vi "sort_property.vi"(6 "Property Order by Default":string[](array[string]), 8 "Sorting Method":u16, 9 "Array to Sort":string[](array[string]), 10 "Property":string[](array[string]), 11 "CmdInfo":T1(array[cluster])=[{"Property"="Arm Slope", "SCPI Command"=":ARM:START:SLOP POS|NEG", "Description"="", "Group"=""}, {"Property"="Arm Enum", "SCPI Command"=":ARM:START:SLOP OK|CANCLE", "Description"="", "Group"=""}]) -> (1 "Sorted Array":string[](array[string]))   [LabVIEW 2018]
doc: "Sort the properties. There are 3 kinds of sorting. When sorting method sets to 0, the properties will be sorted according to their ordir in source command file. When sorting method sets to 1, the properties will be sorted by property names. When sorting method sets to 2, the properties will be sorted by SCPI commands."
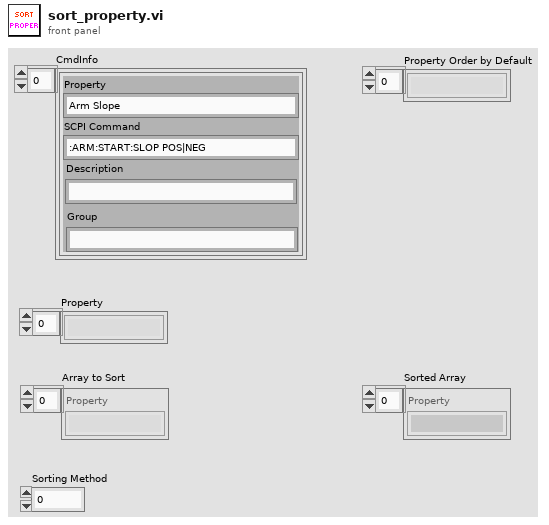
[diagram p1: front panel]
types:
  T1 = cluster{"Property":string, "SCPI Command":string, "Description":string, "Group":string}[]
  T2 = cluster{"SCPI Command":string, "Property":string}[]
  T3 = cluster{"SCPI Command":string, "Property":string}
  T4 = cluster{"Property":string, "SCPI Command":string, "Description":string, "Group":string}
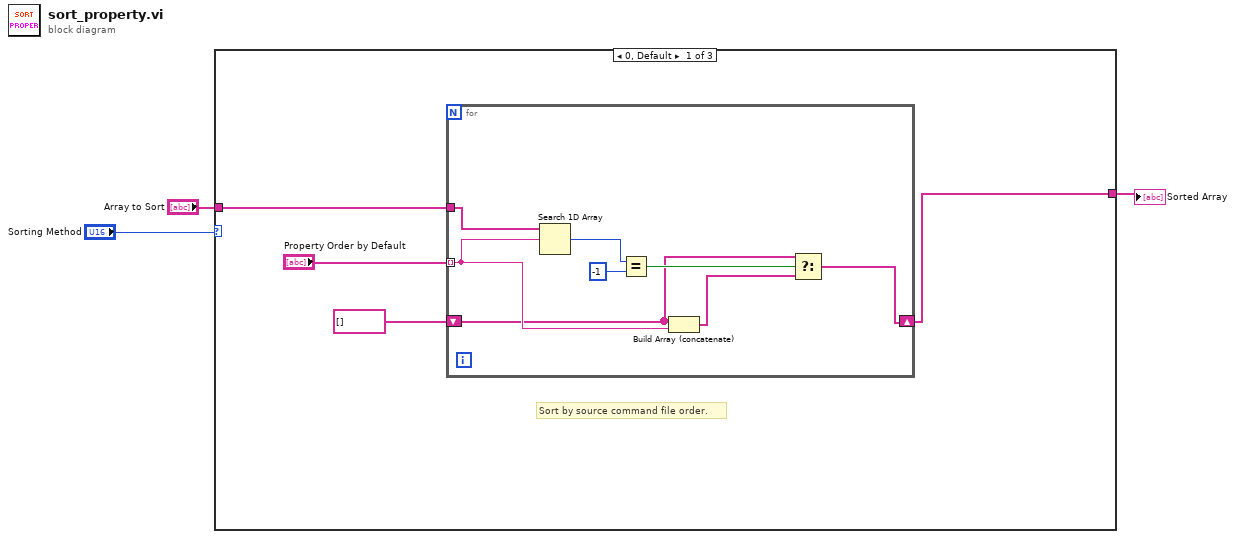
[diagram p0: block diagram]
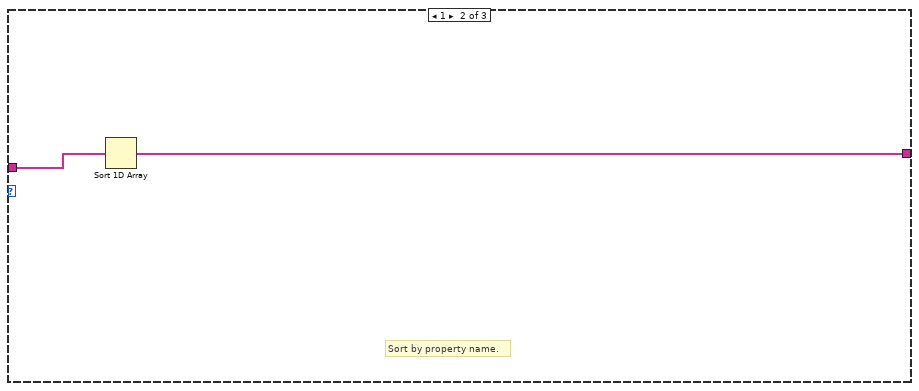
[diagram p2: hidden frame]
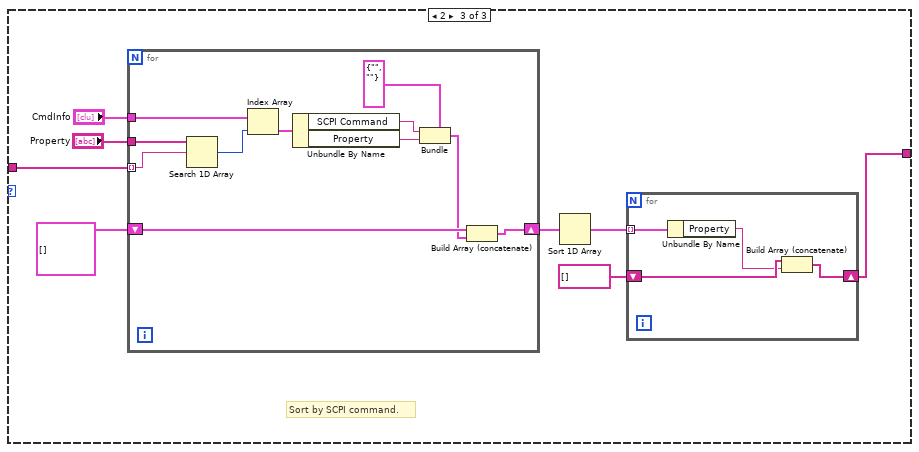
[diagram p3: hidden frame]
diagram:
  n1 = case shown="0, Default" "Sorting Method" {
    tunnel: "Array to Sort" -> [w6 w17 w22]
    tunnel: [w4 w16 w18] -> w1
    frame 0, Default {
      # "Sort by source command file order."
      n2 = for {
        tunnel: "Property Order by Default" -> [w10] mode=indexing
        tunnel: w6 -> [w15]
        shift-right: [w14] -> w4
        shift-left: string[] [] -> [w9]
        n3 = Search 1D Array(1D array=w15, element=w10) -> (index of element=w12:i32)  [unwired: 1 in]
        n4 = Equal?(x=w12, y=-1) -> (x = y?=w11:bool)
        n5 = Build Array (concatenate)(w9, w10) -> (w8:string[])
        n6 = Select(t=w9, s=w11, f=w8) -> (s? t:f=w14:string[])
      }
    }
    frame 1 {
      # "Sort by property name."
      n7 = Sort 1D Array(array=w17) -> (sorted array=w16:string[])
    }
    frame 2 {
      # "Sort by SCPI command."
      n8 = for {
        tunnel: "CmdInfo" -> [w37]
        shift-right: [w30] -> w21
        shift-left: T2 [] ("Array to Sort") -> [w35]
        tunnel: "Property" -> [w39]
        tunnel: w22 -> [w40] mode=indexing
        n9 = Search 1D Array(1D array=w39, element=w40) -> (index of element=w38:i32)  [unwired: 1 in]
        n10 = Index Array(array=w37, index=w38) -> (element=w36:T4)
        n11 = Unbundle By Name(w36) -> ("SCPI Command"=w34:string, "Property"=w33:string)
        n12 = Bundle(cluster=T3 {"SCPI Command"="", "Property"=""}, "SCPI Command"=w34, "Property"=w33) -> (w31:T3)
        n13 = Build Array (concatenate)(w35, w31) -> (w30:T2)
      }
      n14 = Sort 1D Array(array=w21) -> (sorted array=w20:T2)
      n15 = for {
        tunnel: w20 -> [w29] mode=indexing
        shift-right: [w26] -> w18
        shift-left: string[] [] -> [w28]
        n16 = Unbundle By Name(w29) -> ("Property"=w27:string)
        n17 = Build Array (concatenate)(w28, w27) -> (w26:string[])
      }
    }
  }
  "Sorted Array" <- w1
